vi "SetBitfiledValue(U64).vi"(8 "error in (no error)":errorcluster, 9 "bitfield value":u64 format="%.0x", 10 "bitfield caps":T1={"offset"=0, "size"=0, "signed?"=TRUE}, 11 "original value":u64 format="%.0x") -> (0 "error out":errorcluster, 3 "update value":u64)   [LabVIEW 2017, in "Bitfield.lvlib"]
uses:
  Bitfield.lvlib
  BitfieldCaps.ctl
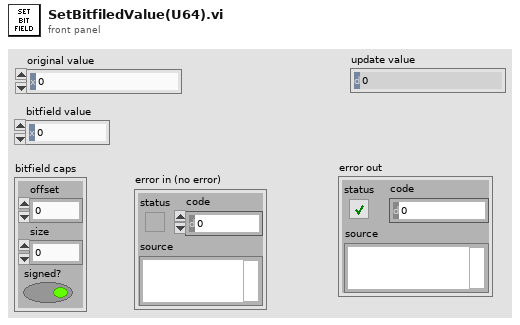
[diagram p1: front panel]
types:
  T1 = typedef "Bitfield.lvlib/BitfieldCaps.ctl" = cluster{"offset":i32, "size":i32, "signed?":bool}
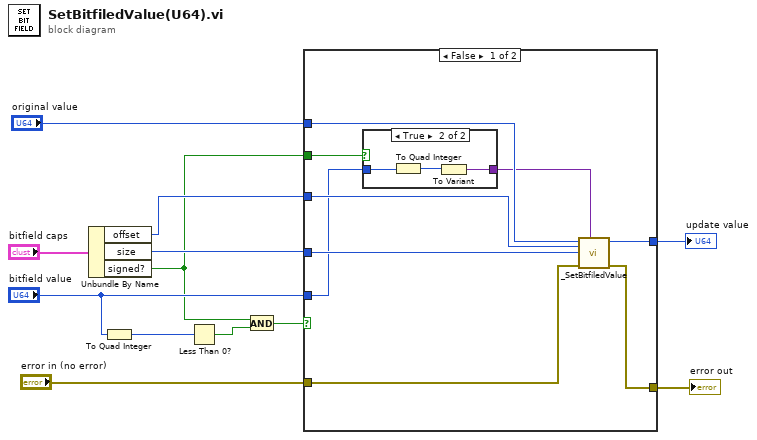
[diagram p0: block diagram]
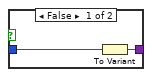
[diagram p2: hidden frame]
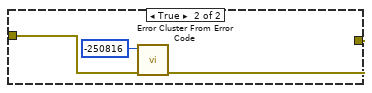
[diagram p3: hidden frame]
diagram:
  n1 = Unbundle By Name("bitfield caps") -> ("offset"=w6:i32, "size"=w5:i32, "signed?"=w1:bool)
  n2 = To Quad Integer(1:"bitfield value") -> (0:w3:i64)
  n3 = Less Than 0?(x=w3) -> (x < 0?=w2:bool)
  n4 = And(x=w1, y=w2) -> (x .and. y?=w12:bool)
  n5 = case shown="False" w12 {
    tunnel: "error in (no error)" -> [w21 w29]
    tunnel: [w19 w27] -> w8
    tunnel: w6 -> [w20 _]
    tunnel: w5 -> [w16 _]
    tunnel: "bitfield value" -> [w14 _]
    tunnel: "original value" -> [w18 _]
    tunnel: [w17 _] -> w9
    tunnel: w1 -> [w15 _]
    frame False {
      n6 = case shown="True" w15 {
        tunnel: w14 -> [w22 w26]
        tunnel: [w23 w24] -> w13
        frame False {
          n7 = To Variant(anything=w22) -> (Variant=w23:variant)
        }
        frame True {
          n8 = To Quad Integer(1:w26) -> (0:w25:i64)
          n9 = To Variant(anything=w25) -> (Variant=w24:variant)
        }
      }
      n10 = call "_SetBitfiledValue.vi"("bitfield value"=w13, "error in (no error)"=w21, "size"=w16, "offset"=w20, "soft value"=w18) -> ("error out"=w19:errorcluster, "update value"=w17:u64)  [unwired: 4 in, 1 out]
    }
    frame True {
      n11 = call <vilib>:"Error Cluster From Error Code.vi"("error in (no error)"=w29, "error code (0)"=-250816) -> ("error out"=w27:errorcluster)  [unwired: 7 in]
    }
  }
  "update value" <- w9
  "error out" <- w8
